vi "Init.vi"(8 "error in (no error)":errorcluster, 11 "Scene Collection Name":string) -> (0 "error out":errorcluster, 3 "SetCurrentSceneCollection out":refnum<class "SetCurrentSceneCollection.lvclass">)   [LabVIEW 2022 SP3, in "obs-websocket-lv.lvlib" / "SetCurrentSceneCollection.lvclass"]
uses:
  SetCurrentSceneCollection.lvclass
  SetCurrentSceneCollection.lvclass/SetCurrentSceneCollection.ctl
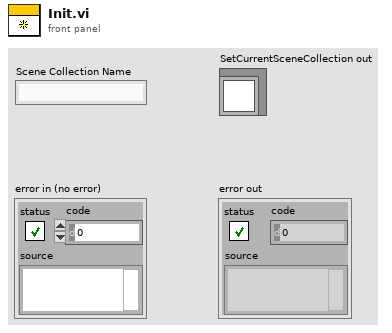
[diagram p1: front panel]
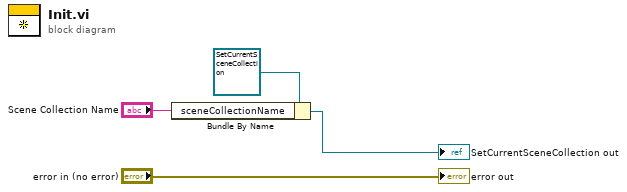
[diagram p0: block diagram]
diagram:
  n1 = Bundle By Name(cluster=refnum<class "SetCurrentSceneCollection.lvclass"> refnum ("SetCurrentSceneCollection in"), "sceneCollectionName"="Scene Collection Name") -> (→"SetCurrentSceneCollection out":refnum<class "SetCurrentSceneCollection.lvclass">)
  "error out" <- "error in (no error)"
